vi "Read calibration config file.vi"(8 "error in (no error)":errorcluster, 11 "configuration file path":path) -> (0 "error out":errorcluster, 3 "Array":cluster{"String":string, string[]}[](array[cluster]))   [LabVIEW 2017]
doc: "Reads a config file and arranges all information into a simple cluster."
uses:
  <vilib>/Utility/config.llb/Read Key (String).vi
  <vilib>/Utility/config.llb/NI_LVConfig.lvlib
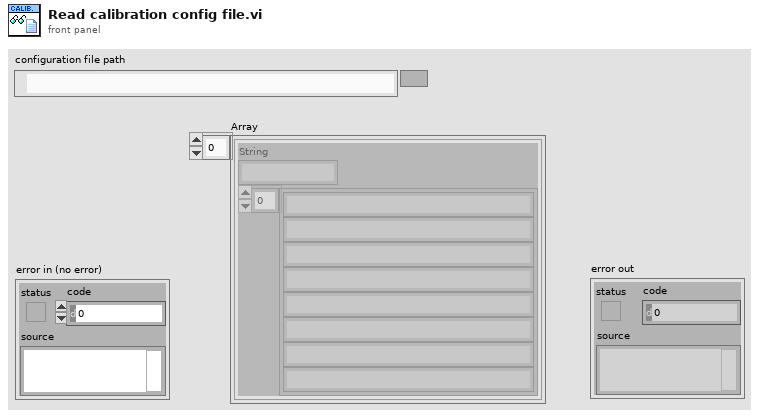
[diagram p1: front panel]
types:
  T1 = typedef "NI_LVConfig.lvlib/Config Data RefNum.ctl" = refnum<k1>
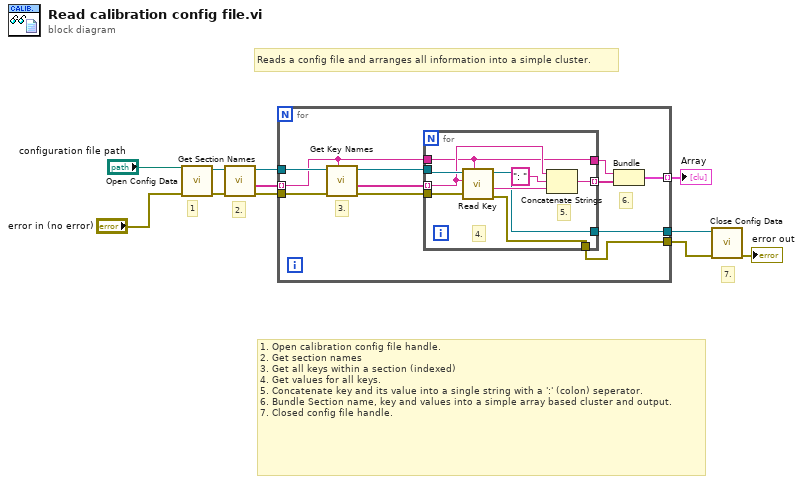
[diagram p0: block diagram]
diagram:
  # "Reads a config file and arranges all information into a simple cluster."
  # "7."
  # "2."
  # "1. Open calibration config file handle.\n2. Get section names\n3. Get all keys within a section (indexed)\n4. Get values for all keys.\n5. Concatenate key and its value into a single string with a ':' (colon) seperator.\n6. Bundle Section name, key and values into a simple array based cluster and output.\n7. Closed config file handle."
  # "1"
  n1 = call <vilib>:"Open Config Data.vi"("error in (no error)"="error in (no error)", "configuration file path"="configuration file path") -> ("error out"=w9:errorcluster, "refnum"=w10:T1)  [unwired: 7 in, 1 out]
  n2 = call <vilib>:"Get Section Names.vi"("error in (no error)"=w9, "refnum"=w10) -> ("error out"=w6:errorcluster, "section names"=w7:string[], "refnum out"=w8:T1)  [unwired: 7 in]
  n3 = for {
    tunnel: w7 -> [w17] mode=indexing
    tunnel: w8 -> [w21]
    tunnel: w6 -> [w22]
    tunnel: [w14] -> w5 mode=indexing
    tunnel: [w13] -> w4
    tunnel: [w12] -> w3
    # "6."
    # "3."
    n4 = call <vilib>:"Get Key Names.vi"("section"=w17, "error in (no error)"=w22, "refnum"=w21) -> ("error out"=w20:errorcluster, "key names"=w18:string[], "refnum out"=w19:T1)  [unwired: 5 in, 1 out]
    n5 = for {
      tunnel: w20 -> [w31]
      tunnel: w19 -> [w30]
      tunnel: w18 -> [w27] mode=indexing
      tunnel: w17 -> [w25]
      tunnel: [w26] -> w16 mode=indexing
      tunnel: [w25] -> w15
      tunnel: [w24] -> w13
      tunnel: [w23] -> w12
      # "5."
      # "4."
      n6 = call-poly <vilib>:"Read Key.vi"("section"=w25, "error in (no error)"=w31, "key"=w27, "refnum"=w30) -> ("error out"=w23:errorcluster, "value"=w29:string, "refnum out"=w24:T1)  [unwired: 4 in, 1 out]
      n7 = Concatenate Strings(w27, ": ", w29) -> (w26:string)
    }
    n8 = Bundle("String"=w15, w16) -> (w14:cluster{"String":string, string[]})  [unwired: 1 in]
  }
  "Array" <- w5
  n9 = call <vilib>:"Close Config Data.vi"("error in (no error)"=w3, "refnum"=w4) -> ("error out"=→"error out":errorcluster)  [unwired: 8 in, 1 out]
